vi "createSerialProtocol.vi"(8 "error in (no error)":errorcluster, 10 "Serial Protocol":T1, 11 "ISerialCommFactory in":refnum<class "ISerialProtocolFactory.lvclass">) -> (0 "error out":errorcluster, 2 "serialProtocol":refnum<class "SerialProtocol.lvclass">, 3 "ISerialCommFactory out":refnum<class "ISerialProtocolFactory.lvclass">)   [LabVIEW 2013, in "SerialProtocols.lvlib" / "ISerialProtocolFactory.lvclass"]
uses:
  <userlib>/Common/SerialProtocols/SerialProtocolFactory/ISerialProtocolFactory/ISerialProtocolFactory.lvclass
  <userlib>/Common/SerialProtocols/SerialProtocol/SerialProtocol/SerialProtocol.lvclass
  <userlib>/Common/SerialProtocols/Configuration/SerialProtocol.ctl
  <userlib>/Common/SerialProtocols/SerialProtocols.lvlib
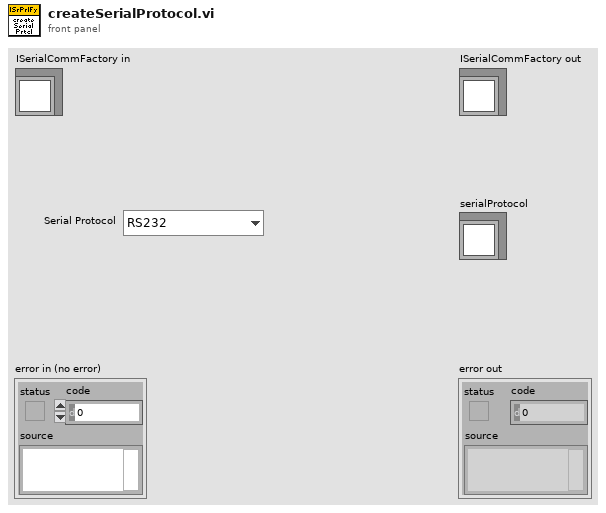
[diagram p1: front panel]
types:
  T1 = typedef "SerialProtocols.lvlib/SerialProtocol.ctl" = enum16{"RS232", "RS485", "SerialSimulator"}
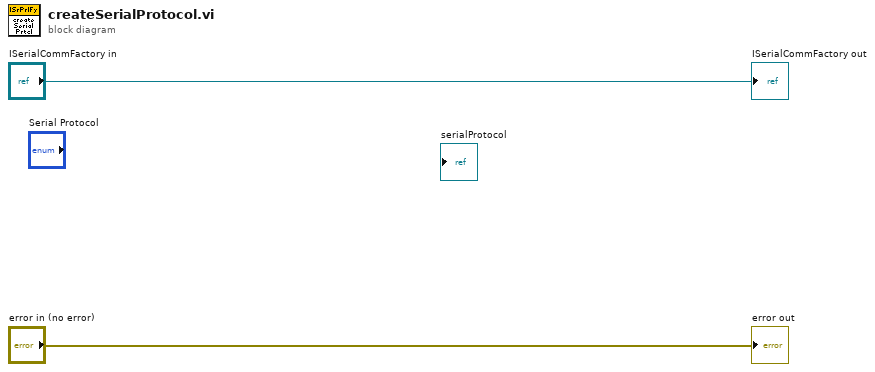
[diagram p0: block diagram]
diagram:
  "error out" <- "error in (no error)"
  "ISerialCommFactory out" <- "ISerialCommFactory in"
